vi "Read Location.vi"(8 "error in (no error)":errorcluster, 11 "Add Metadata Msg in":refnum<class "Add Metadata Msg.lvclass">) -> (0 "error out":errorcluster, 2 "Location":string, 3 "Add Metadata Msg out":refnum<class "Add Metadata Msg.lvclass">)   [LabVIEW 2021, in "Add Metadata Msg.lvclass"]
uses:
  Add Metadata Msg.lvclass
  Add Metadata Msg.lvclass/Add Metadata Msg.ctl
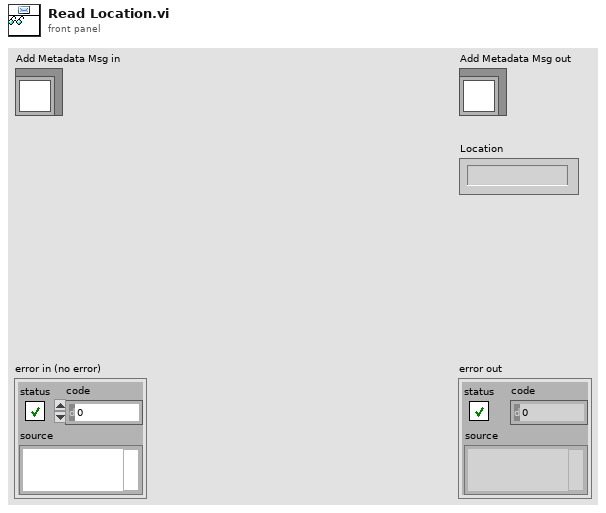
[diagram p1: front panel]
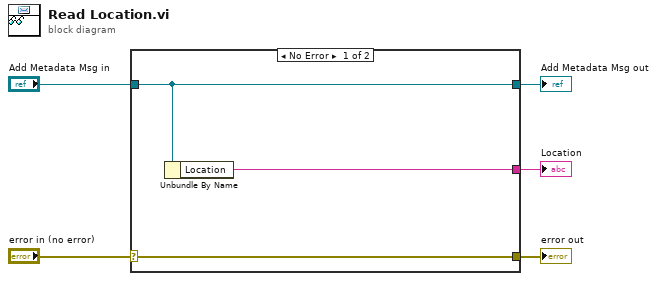
[diagram p0: block diagram]
diagram:
  n1 = case shown="No Error" "error in (no error)" {
    selector: "error in (no error)" -> [w8 w9]
    tunnel: [w8 w9] -> w4
    tunnel: [w7 w10] -> w2
    tunnel: "Add Metadata Msg in" -> [w7 w10]
    tunnel: [w6 _] -> w1
    frame No Error {
      n2 = Unbundle By Name(w7) -> ("Location"=w6:string)
    }
    frame Error {
    }
  }
  "error out" <- w4
  "Add Metadata Msg out" <- w2
  "Location" <- w1
